vi "Stream Low Latency.vi"() -> ()   [LabVIEW 2020]
panel:
  in  "#Seconds on Graph":dbl=1.0 format="%.2f"
  out "Actual SampleRate (Hz)":dbl format="%.3f"
  out "NumAddresses":i32
  in  "STREAM_RESOLUTION_INDEX":i32
  in  "STREAM_SETTLING_US":i32
  in  "AIN_ALL_RANGE":dbl=10.0 format="%.3f"
  out "ScansPerRead":i32
  out "ConnectionType Out":i32
  out "DeviceType Out":i32
  in  "Identifier":string="LJM_idANY"
  in  "ConnectionType":string="LJM_ctANY"
  in  "DeviceType":string="LJM_dtANY"
  out "DeviceScanBacklog":i32
  out "LJMScanBacklog":i32
  out "Data":dbl[][](array[numeric]) format="%.3f"
  out "Waveform Graph":dbl[][](graph)
  in  "Scan List":string[](array[string])=["AIN0", "AIN1", "AIN2", "AIN3"]
  out "# of iterations":i32
  in  "Scan Rate (Hz)":dbl=1000.0 format="%.3f"
  in  "stop":bool
  out "Error Message":string
  # "To remove an element, right-click\non it, select Data Operations =>\nRemove Element.\n\nTo empty an array, right-click\nnear the edge, select Data\nOperations => Empty Array.\n\nOther useful operations:  From the\nOperate menu are \"Make Current\nValues Default\" and \"Reinitialize\nTo Default\"."
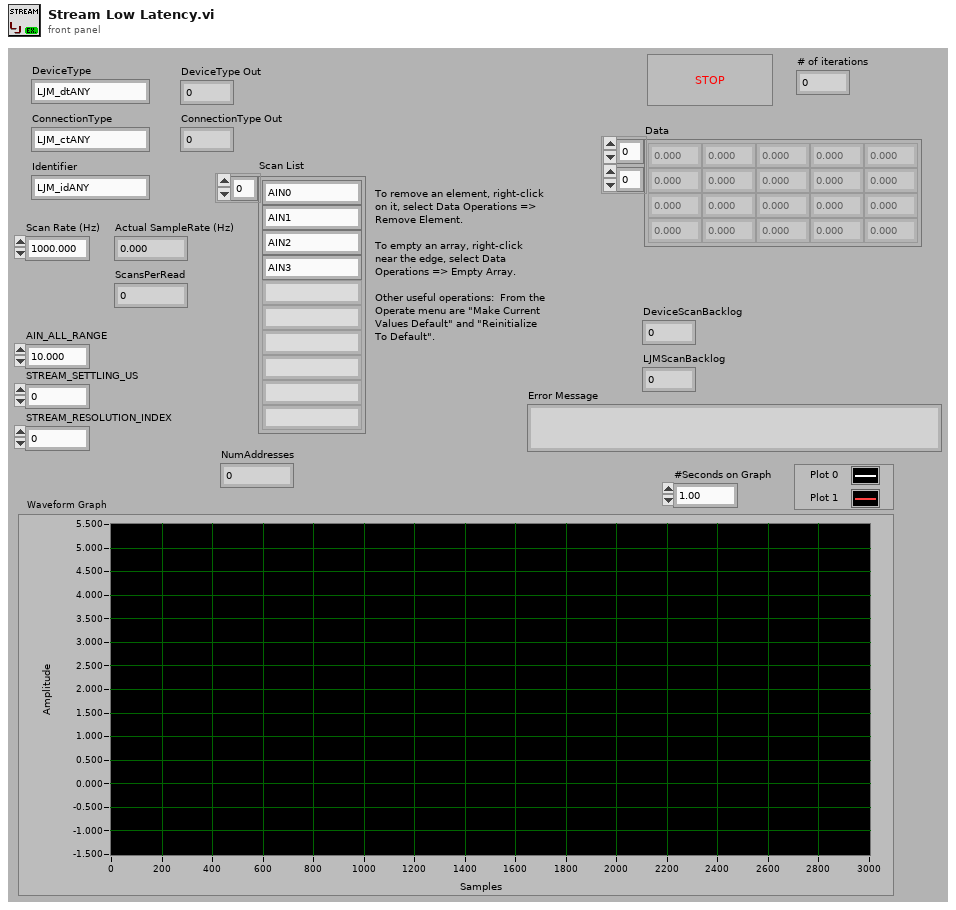
[diagram p1: front panel]
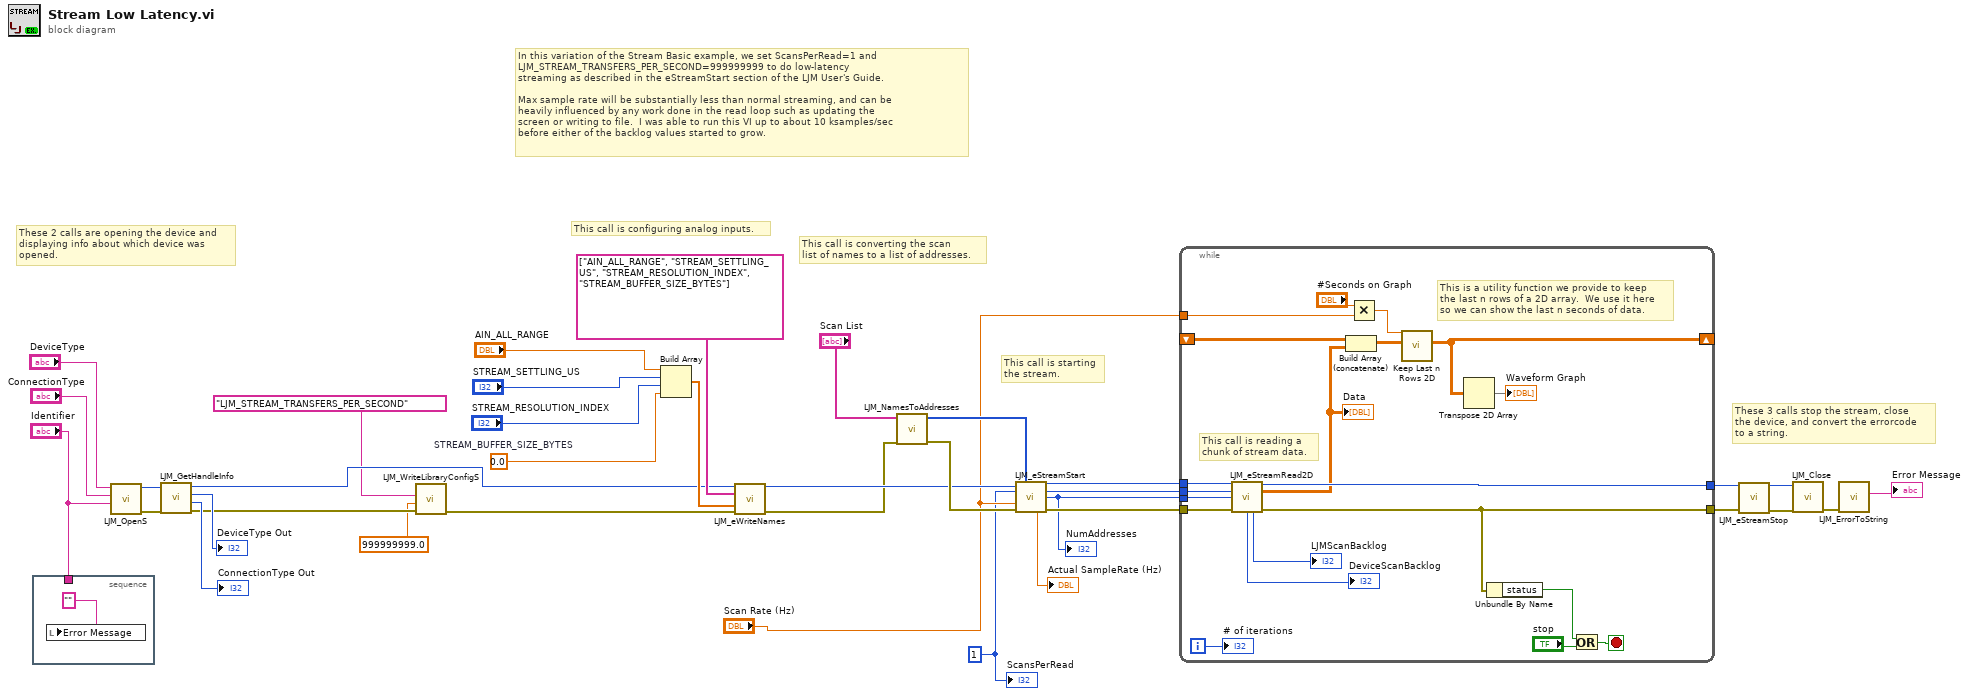
[diagram p0: block diagram]
diagram:
  w6 = 1
  w8 = 0.0  # STREAM_BUFFER_SIZE_BYTES
  # "In this variation of the Stream Basic example, we set ScansPerRead=1 and\nLJM_STREAM_TRANSFERS_PER_SECOND=999999999 to do low-latency\nstreaming as described in the eStreamStart section of the LJM User's Guide.\n\nMax sample rate will be substantially less than normal streaming, and can be\nheavily influenced by any work done in the read loop such as updating the\nscreen or writing to file.  I was able to run this VI up to about 10 ksamples/sec\nbefore either of the backlog values started to grow."
  # "These 3 calls stop the stream, close\nthe device, and convert the errorcode\nto a string."
  # "This call is starting\nthe stream."
  # "This call is converting the scan\nlist of names to a list of addresses."
  # "This call is configuring analog inputs."
  # "These 2 calls are opening the device and\ndisplaying info about which device was\nopened."
  n1 = stacked-sequence {
    tunnel: "Identifier" -> [_]
    frame #0 {
      n2 = local write "Error Message"("" ("Error Message")) -> ()
    }
  }
  n3 = call "LJM_OpenS.vi"("Identifier"="Identifier", "ConnectionType"="ConnectionType", "DeviceType"="DeviceType") -> ("error out"=w28:errorcluster, "Handle"=w25:i32)  [unwired: 7 in]
  n4 = call "LJM_GetHandleInfo.vi"("error in"=w28, "Handle In"=w25) -> ("error out"=w5:errorcluster, "ConnectionType"=→"ConnectionType Out":i32, "DeviceType"=→"DeviceType Out":i32, "Handle Out"=w3:i32)  [unwired: 2 in, 4 out]
  n5 = call "LJM_WriteLibraryConfigS.vi"("error in"=w5, "Value"=999999999.0, "Parameter"="LJM_STREAM_TRANSFERS_PER_SECOND") -> ("error out"=w4:errorcluster)  [unwired: 8 in]
  n6 = Build Array("AIN_ALL_RANGE", "STREAM_SETTLING_US", "STREAM_RESOLUTION_INDEX", w8) -> (w16:dbl[])
  n7 = call "LJM_eWriteNames.vi"("Handle In"=w3, "aNames"=string[] ["AIN_ALL_RANGE", "STREAM_SETTLING_US", "STREAM_RESOLUTION_INDEX", "STREAM_BUFFER_SIZE_BYTES"], "aValuesIn"=w16, "error in"=w4) -> ("Handle Out"=w20:i32, "error out"=w19:errorcluster)  [unwired: 9 in, 1 out]
  n8 = call "LJM_NamesToAddresses.vi"("error in"=w19, "aNames"="Scan List") -> ("error out"=w21:errorcluster, "aAddresses"=w13:i32[])  [unwired: 7 in, 1 out]
  n9 = call "LJM_eStreamStart.vi"("Handle In"=w20, "aScanList"=w13, "ScansPerRead"=w6, "ScanRate"="Scan Rate (Hz)", "error in"=w21) -> ("Handle Out"=w35:i32, "ScansPerRead Out"=w9:i32, "NumReadAddresses"=w11:i32, "Actual SampleRate"=→"Actual SampleRate (Hz)":dbl, "error out"=w36:errorcluster)  [unwired: 5 in, 1 out]
  "NumAddresses" <- w11
  n10 = while {
    tunnel: [w51] -> w33
    tunnel: w35 -> [w52]
    tunnel: w11 -> [w47]
    tunnel: w9 -> [w46]
    shift-right: [w38] -> _
    shift-left: _ -> [w43]
    tunnel: "Scan Rate (Hz)" -> [w41]
    tunnel: w36 -> [w53]
    tunnel: [w48] -> w34
    i -> [w54]
    stop <- w55 stop-if-true
    # "This call is reading a\nchunk of stream data."
    # "This is a utility function we provide to keep\nthe last n rows of a 2D array.  We use it here\nso we can show the last n seconds of data."
    n11 = call "LJM_eStreamRead2D.vi"("Handle In"=w52, "ScansPerRead"=w46, "NumAddresses"=w47, "error in"=w53) -> ("Handle Out"=w51:i32, "aData Out"=w42:dbl[][], "DeviceScanBacklog"=→"DeviceScanBacklog":i32, "LJMScanBacklog"=→"LJMScanBacklog":i32, "error out"=w48:errorcluster)  [unwired: 7 in]
    "Data" <- w42
    n12 = Build Array (concatenate)(w43, w42) -> (w40:dbl[][])
    n13 = Multiply(x="#Seconds on Graph", y=w41) -> (x*y=w39:dbl)
    n14 = call "Keep Last n Rows 2D.vi"("Array"=w40, "# Rows to Keep"=w39) -> ("Last n Rows"=w38:dbl[][])  [unwired: 9 in]
    n15 = Transpose 2D Array(2D array=w38) -> (transposed array=→"Waveform Graph":dbl[][])
    n16 = Unbundle By Name(w48) -> ("status"=w56:bool)
    n17 = Or(x=w56, y="stop") -> (x .or. y?=w55:bool)
    "# of iterations" <- w54
  }
  n18 = call "LJM_eStreamStop.vi"("Handle In"=w33, "error in"=w34) -> ("Handle Out"=w31:i32, "error out"=w32:errorcluster)  [unwired: 12 in]
  n19 = call "LJM_Close.vi"("error in"=w32, "Handle"=w31) -> ("error out"=w30:errorcluster)  [unwired: 9 in]
  n20 = call "LJM_ErrorToString.vi"("error in"=w30) -> ("String"=→"Error Message":string)  [unwired: 10 in]
  "ScansPerRead" <- w6
